vi "Write.vi"(7 "Wait Until Done?":bool, 8 "error in (no error)":errorcluster, 9 "Sample Rate [Hz]":dbl=1000.0 min=1000.0 max=8000000.0, 10 "Values":bool[][](array[boolean]), 11 "DO (N Samples) Ref In":T1) -> (0 "error out":errorcluster, 3 "DO (N Samples) Ref Out":T1)   [LabVIEW 2021, in "DO Block.lvlib"]
doc: "Writes values to one or more digital output channels. Use this VI to write multiple samples for each channel at one time."
uses:
  <vilib>/myRIO/Instrument Drivers/Onboard IO/DO Block/DO Block.lvlib
  <vilib>/myRIO/Instrument Drivers/Onboard IO/DO Block/typedefs/DO Block Reference.ctl
  <vilib>/myRIO/Common/Instrument Driver Framework/Utilities/typedefs/myRIO Generic Hardware Reference.ctl
  <vilib>/myRIO/Common/Instrument Driver Framework/Utilities/typedefs/Hardware Version Enum.ctl
  <vilib>/myRIO/Common/Instrument Driver Framework/Utilities/typedefs/myRIO v1.0 Reference.ctl
  <vilib>/myRIO/Common/Instrument Driver Framework/Utilities/typedefs/Generic FPGA Reference.ctl
  <vilib>/myRIO/Common/Instrument Driver Framework/myRIO v1.0/DO Block/typedefs/DO Block Channels List.ctl
  <vilib>/myRIO/Common/Instrument Driver Framework/myRIO v1.0/DO Block/typedefs/DO Block Channels Enum.ctl
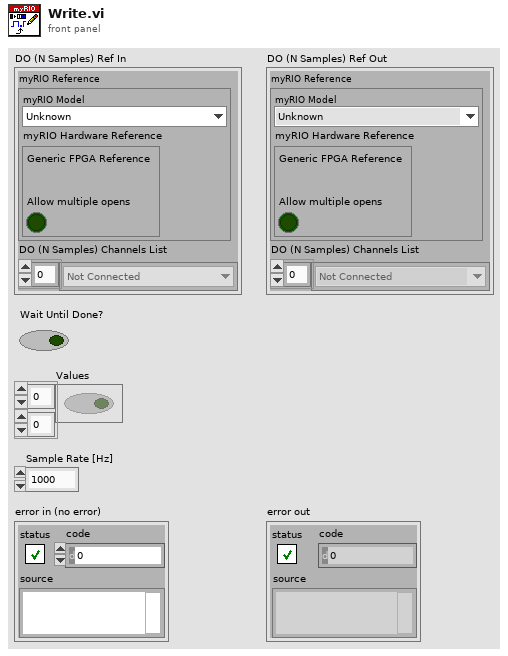
[diagram p1: front panel]
types:
  T1 = typedef "DO Block.lvlib/DO Block Reference.ctl" = cluster{"myRIO Reference":T2, "DO (N Samples) Channels List":T6}
  T2 = typedef "myRIO Generic Hardware Reference.ctl" = cluster{"myRIO Model":T3, "myRIO Hardware Reference":T4}
  T3 = typedef "Hardware Version Enum.ctl" = enum16{"Unknown", "myRIO-1900", "myRIO-1950", "roboRIO", "NI ELVIS RIO CM", "ELVIS III"}
  T4 = typedef "myRIO v1.0 Reference.ctl" = cluster{"Generic FPGA Reference":T5, "Allow multiple opens":bool}
  T5 = typedef "Generic FPGA Reference.ctl" = refnum<k20>
  T6 = typedef "DO Block Channels List.ctl" = T7[]
  T7 = typedef "DO Block Channels Enum.ctl" = enum16{"Not Connected", "A/DO0 (N Samples)", "A/DO1 (N Samples)", "A/DO2 (N Samples)", "A/DO3 (N Samples)", "A/DO4 (N Samples)", "A/DO5 (N Samples)", "A/DO6 (N Samples)", "A/DO7 (N Samples)", "A/DO8 (N Samples)", "A/DO9 (N Samples)", "A/DO10 (N Samples)", "A/DO11 (N Samples)", "A/DO12 (N Samples)", "A/DO13 (N Samples)", "A/DO14 (N Samples)", "A/DO15 (N Samples)", "A/DO16 (N Samples)", "A/DO17 (N Samples)", "A/DO18 (N Samples)", "A/DO19 (N Samples)", "B/DO0 (N Samples)", "B/DO1 (N Samples)", "B/DO2 (N Samples)", "B/DO3 (N Samples)", "B/DO4 (N Samples)", "B/DO5 (N Samples)", "B/DO6 (N Samples)", "B/DO7 (N Samples)", "B/DO8 (N Samples)", "B/DO9 (N Samples)", "B/DO10 (N Samples)", "B/DO11 (N Samples)", "B/DO12 (N Samples)", "B/DO13 (N Samples)", "B/DO14 (N Samples)", "B/DO15 (N Samples)", "B/DO16 (N Samples)", "B/DO17 (N Samples)", "B/DO18 (N Samples)", "B/DO19 (N Samples)"}
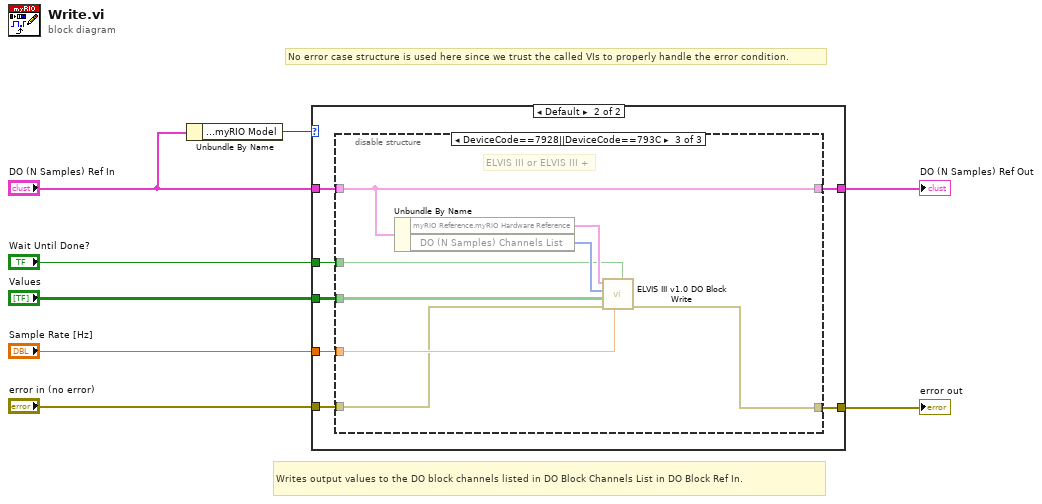
[diagram p0: block diagram]
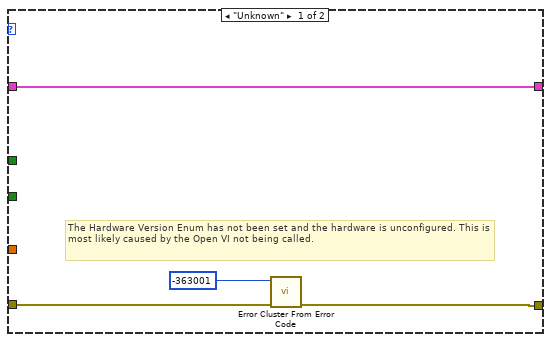
[diagram p2: hidden frame]
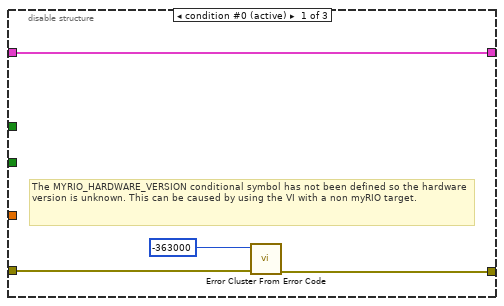
[diagram p3: hidden frame]
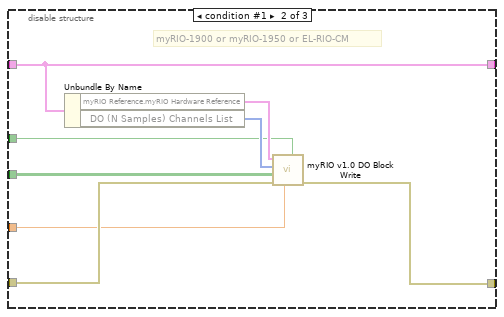
[diagram p4: hidden frame]
diagram:
  # "No error case structure is used here since we trust the called VIs to properly handle the error condition."
  # "Writes output values to the DO block channels listed in DO Block Channels List in DO Block Ref In."
  n1 = Unbundle By Name("DO (N Samples) Ref In") -> ("myRIO Reference.myRIO Model"=w3:T3)
  n2 = case shown="Default" w3 {
    tunnel: [w11 w19] -> w5
    tunnel: "DO (N Samples) Ref In" -> [w9 w18]
    tunnel: "error in (no error)" -> [w10 w17]
    tunnel: [w9 w16] -> w6
    tunnel: "Values" -> [_ w15]
    tunnel: "Sample Rate [Hz]" -> [_ w14]
    tunnel: "Wait Until Done?" -> [_ w13]
    frame "Unknown" {
      # "The Hardware Version Enum has not been set and the hardware is unconfigured. This is most likely caused by the Open VI not being called."
      n3 = call <vilib>:"Error Cluster From Error Code.vi"("error in (no error)"=w10, "error code (0)"=-363001) -> ("error out"=w11:errorcluster)  [unwired: 7 in]
    }
    frame Default {
      n4 = disable-structure shown="DeviceCode==7928||DeviceCode==793C" {
        disable-tunnel: w18 -> [w20 w26 w37]
        disable-tunnel: [w23 w29 w36] -> w19
        disable-tunnel: w17 -> [w21 w31 w32]
        disable-tunnel: [w20 w26 w37] -> w16
        disable-tunnel: w15 -> [_ w27 w35]
        disable-tunnel: w14 -> [_ w24 w33]
        disable-tunnel: w13 -> [_ w25 w34]
        frame condition #0 (active) {
          # "The MYRIO_HARDWARE_VERSION conditional symbol has not been defined so the hardware version is unknown. This can be caused by using the VI with a non myRIO target."
          n5 = call <vilib>:"Error Cluster From Error Code.vi"("error in (no error)"=w21, "error code (0)"=-363000) -> ("error out"=w23:errorcluster)  [unwired: 7 in]
        }
        frame condition #1 {
          # "myRIO-1900 or myRIO-1950 or EL-RIO-CM"
          n6 = Unbundle By Name(w26) -> ("myRIO Reference.myRIO Hardware Reference"=w28:T4, "DO (N Samples) Channels List"=w30:T6)
          n7 = call <vilib>:"myRIO v1.0 DO Block Write.vi"("Wait Until Done?"=w25, "DO FIFO Sample Rate (Hz)"=w24, "error in (no error)"=w31, "bool Value List"=w27, "DO (N Samples) Channel List"=w30, "myRIO Ref In"=w28) -> ("error out"=w29:errorcluster)  [unwired: 4 in, 1 out]
        }
        frame condition #2 {
          # "ELVIS III or ELVIS III +"
          n8 = Unbundle By Name(w37) -> ("myRIO Reference.myRIO Hardware Reference"=w38:T4, "DO (N Samples) Channels List"=w39:T6)
          n9 = call <vilib>:"ELVIS III v1.0 DO Block Write.vi"("Wait Until Done?"=w34, "DO FIFO Sample Rate (Hz)"=w33, "error in (no error)"=w32, "Data by Channel"=w35, "DO (N Samples) Channel List"=w39, "myRIO Ref In"=w38) -> ("error out"=w36:errorcluster)  [unwired: 4 in, 1 out]
        }
      }
    }
  }
  "DO (N Samples) Ref Out" <- w6
  "error out" <- w5
